vi "createTuplaEnDBVarilla.vi"(8 "error in":errorcluster, 11 "claseVarilla in":refnum<class "claseVarilla.lvclass">) -> (0 "error out":errorcluster, 3 "claseVarilla out":refnum<class "claseVarilla.lvclass">)   [LabVIEW 2014, in "claseVarilla.lvclass"]
uses:
  claseVarilla.lvclass
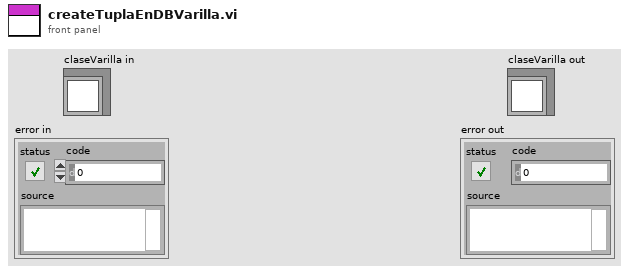
[diagram p1: front panel]
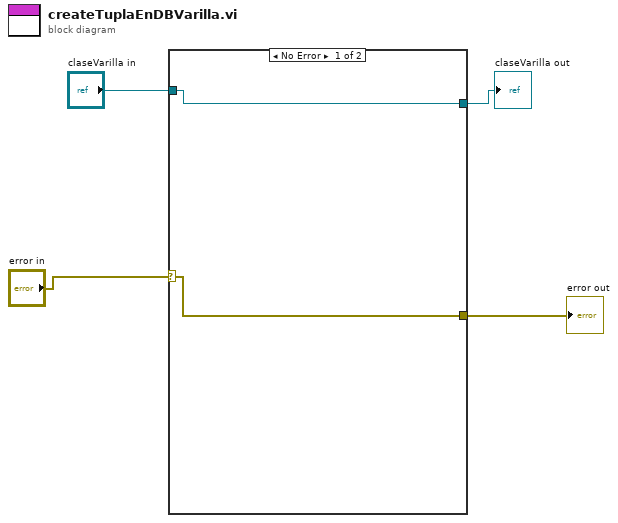
[diagram p0: block diagram]
diagram:
  n1 = case shown="No Error" "error in" {
    selector: "error in" -> [w6 w8]
    tunnel: [w6 w8] -> w3
    tunnel: [w5 w7] -> w2
    tunnel: "claseVarilla in" -> [w5 w7]
    frame No Error {
    }
    frame Error {
    }
  }
  "claseVarilla out" <- w2
  "error out" <- w3
